vi "Laurel Meter Serial.vi"(8 "error in (no error)":errorcluster, 10 "VISA Input":refnum<visa-resource-name>, 11 "Laurel Serial Commands":T1) -> (0 "error out":errorcluster, 2 "VISA Output":refnum<visa-resource-name>, 3 "Output":dbl format="%.2f")   [LabVIEW 2019]
uses:
  Type Definitions/Laurel Serial Commands.ctl
  <vilib>/Utility/error.llb/whitespace.ctl
panel:
  out "length":i32
  in  "All Active byte count":u32=16
  in  "byte count":u32=9
  out "Send Command":string
  out "return count":u32
  out "read buffer":string
  # "Laurel Meter Setup"
  # "Ethernet"
  # "Power Input"
  # "Item 2"
  # "Manual\nReset"
  # "Item 1"
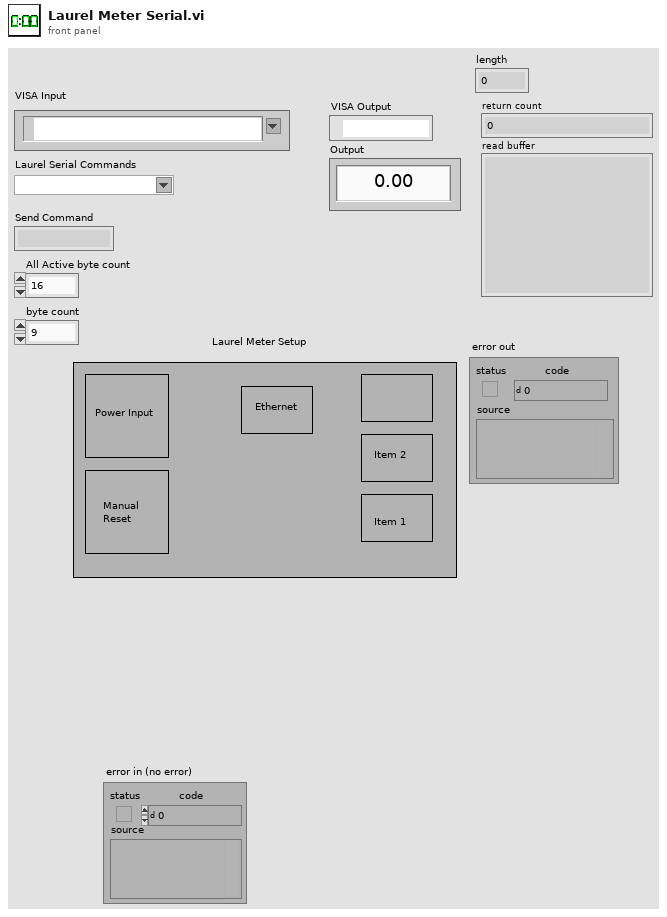
[diagram p1: front panel]
types:
  T1 = typedef "Laurel Serial Commands.ctl" = string
  T2 = typedef "whitespace.ctl" = u16
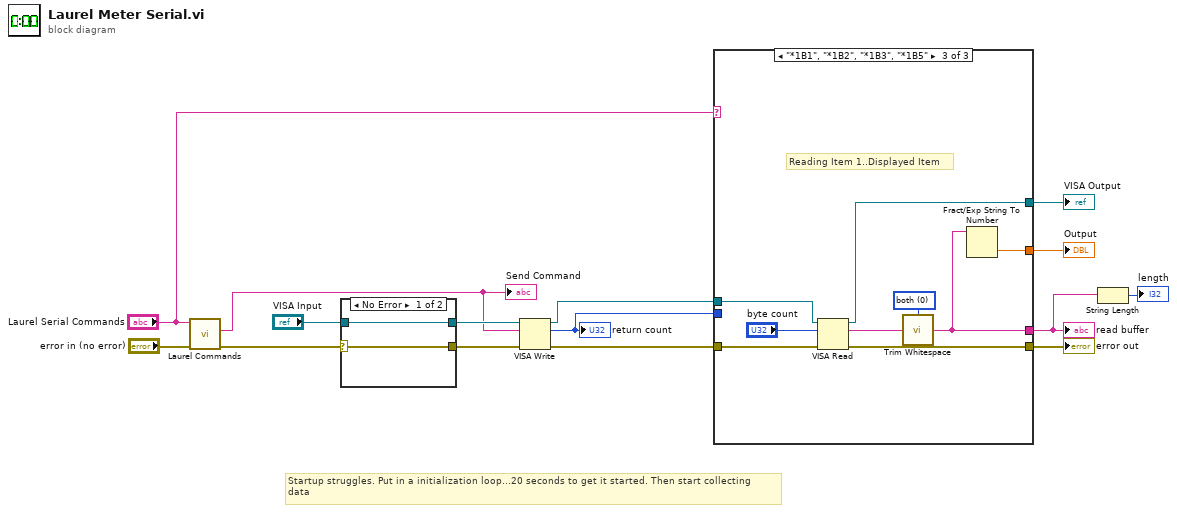
[diagram p0: block diagram]
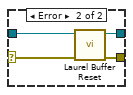
[diagram p2: hidden frame]
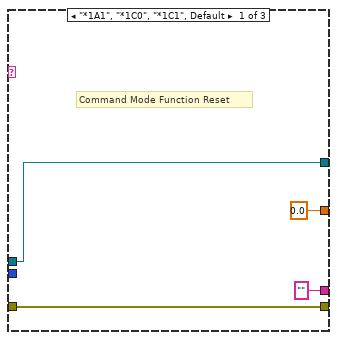
[diagram p3: hidden frame]
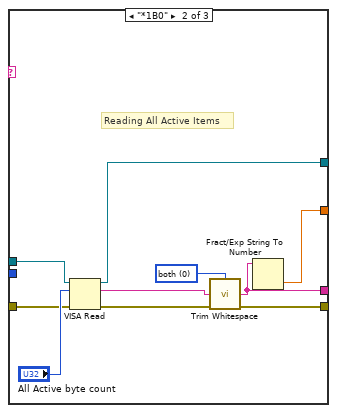
[diagram p4: hidden frame]
diagram:
  # "Startup struggles. Put in a initialization loop...20 seconds to get it started. Then start collecting\ndata"
  n1 = call "Laurel Commands.vi"("Error In"="error in (no error)", "Laurel Serial Commands"="Laurel Serial Commands") -> ("Error Out"=w4:errorcluster, "Send Command out"=w6:string)  [unwired: 8 in]
  "Send Command" <- w6
  n2 = case shown="No Error" w4 {
    selector: w4 -> [w17 w19]
    tunnel: "VISA Input" -> [w16 w18]
    tunnel: [w16 w21] -> w8
    tunnel: [w17 w20] -> w12
    frame No Error {
    }
    frame Error {
      n3 = call "Laurel Buffer Reset.vi"("error in (no error)"=w19, "VISA Refnum in"=w18) -> ("error out"=w20:errorcluster, "VISA Refnum out"=w21:refnum<visa-resource-name>)  [unwired: 8 in]
    }
  }
  n4 = VISA Write(VISA resource name=w8, write buffer=w6, error in (no error)=w12) -> (VISA resource name out=w15:refnum<visa-resource-name>, return count=w11:u32, error out=w7:errorcluster)
  "return count" <- w11
  n5 = case shown="\"*1B1\", \"*1B2\", \"*1B3\", \"*1B5\"" "Laurel Serial Commands" {
    tunnel: w15 -> [w25 w31 w43]
    tunnel: [w22 w34 w41] -> w10
    tunnel: [w25 w33 w42] -> w14
    tunnel: [0.0 w30 w40] -> w9
    tunnel: ["" ("read buffer") w28 w38] -> w2
    tunnel: w11 -> [_ _ _]
    tunnel: w7 -> [w22 w26 w35]
    frame "*1A1", "*1C0", "*1C1", Default {
      # "Command Mode Function Reset"
    }
    frame "*1B0" {
      w27 = T2 0 items=["both", "start of string", "end of string"] ("location (both)")
      # "Reading All Active Items"
      n6 = VISA Read(VISA resource name=w31, byte count="All Active byte count", error in (no error)=w26) -> (VISA resource name out=w33:refnum<visa-resource-name>, read buffer=w29:string, error out=w34:errorcluster)  [unwired: 1 out]
      n7 = call <vilib>:"Trim Whitespace.vi"("string"=w29, "location (both)"=w27) -> ("trimmed string"=w28:string)
      n8 = Fract/Exp String To Number(string=w28) -> (number=w30:dbl)  [unwired: 3 in, 1 out]
    }
    frame "*1B1", "*1B2", "*1B3", "*1B5" {
      w37 = T2 0 items=["both", "start of string", "end of string"] ("location (both)")
      # "Reading Item 1..Displayed Item"
      n9 = VISA Read(VISA resource name=w43, byte count="byte count", error in (no error)=w35) -> (VISA resource name out=w42:refnum<visa-resource-name>, read buffer=w39:string, error out=w41:errorcluster)  [unwired: 1 out]
      n10 = call <vilib>:"Trim Whitespace.vi"("string"=w39, "location (both)"=w37) -> ("trimmed string"=w38:string)
      n11 = Fract/Exp String To Number(string=w38) -> (number=w40:dbl)  [unwired: 3 in, 1 out]
    }
  }
  "error out" <- w10
  "VISA Output" <- w14
  "read buffer" <- w2
  "Output" <- w9
  n12 = String Length(string=w2) -> (length=→"length":i32)
